vi "Get_FileToLoad.vi"(8 "error in (no error)":errorcluster, 11 "ExampleStateMachine runtime_in":refnum<class "ExampleStateMachine runtime.lvclass">) -> (0 "error out":errorcluster, 2 "FileToLoad":path, 3 "ExampleStateMachine runtime_out":refnum<class "ExampleStateMachine runtime.lvclass">)   [LabVIEW 2017, in "ExampleStateMachine runtime.lvclass"]
uses:
  ExampleStateMachine runtime.lvclass
  ExampleStateMachine runtime.lvclass/ExampleStateMachine runtime.ctl
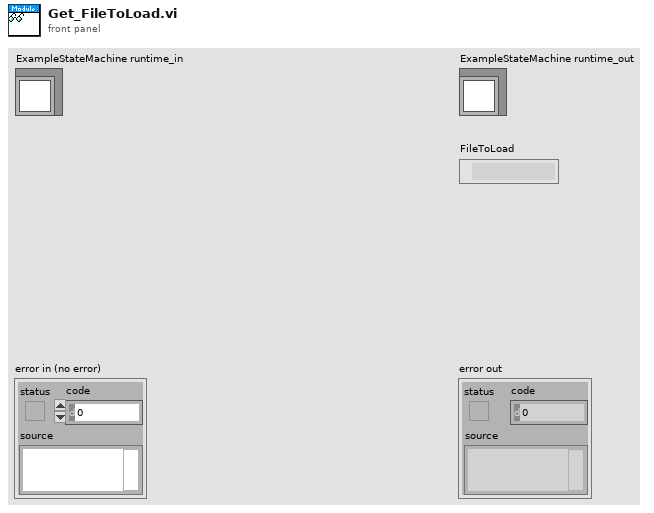
[diagram p1: front panel]
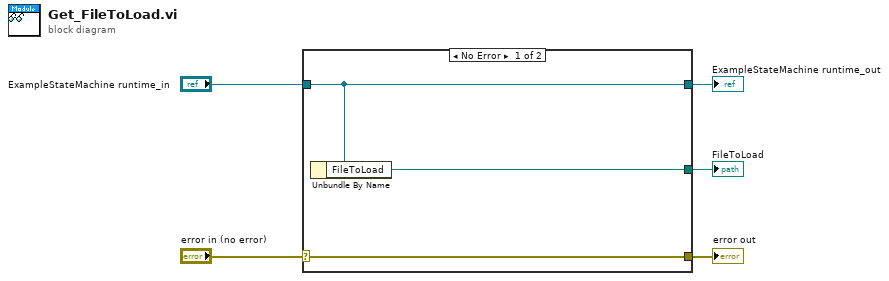
[diagram p0: block diagram]
diagram:
  n1 = case shown="No Error" "error in (no error)" {
    selector: "error in (no error)" -> [w8 w9]
    tunnel: [w8 w9] -> w4
    tunnel: [w7 w10] -> w2
    tunnel: "ExampleStateMachine runtime_in" -> [w7 w10]
    tunnel: [w6 _] -> w1
    frame No Error {
      n2 = Unbundle By Name(w7) -> ("FileToLoad"=w6:path)
    }
    frame Error {
    }
  }
  "error out" <- w4
  "ExampleStateMachine runtime_out" <- w2
  "FileToLoad" <- w1
